vi "Fundamental Power Values (1 Cycle).vi"(0 "one-cycle fundamental phase voltage vectors":T3(array[cluster]), 5 "one-cycle fundamental current vectors":T3(array[cluster]), 9 "system info in":refnum<class "EP System Info.lvclass">, 11 "error in (no error)":errorcluster) -> (4 "one-cycle fundamental power values":T1(array[cluster]), 10 "system info out":refnum<class "EP System Info.lvclass">, 15 "error out":errorcluster)   [LabVIEW 2014, in "NI_EP_Power Quality.lvlib"]
doc: "Calculates the fundamental power values from the voltage and current spectra for a single-cycle block.\n\nThis VI supports measuring single-line and multiple-line systems."
uses:
  <vilib>/addons/Electrical Power/PQ/NI_EP_Power Quality.lvlib
  <vilib>/addons/Electrical Power/PQ/Common/Controls/ep_AI Data Channel.ctl
  <vilib>/addons/Electrical Power/PQ/Common/Classes/System Info/EP System Info.lvclass
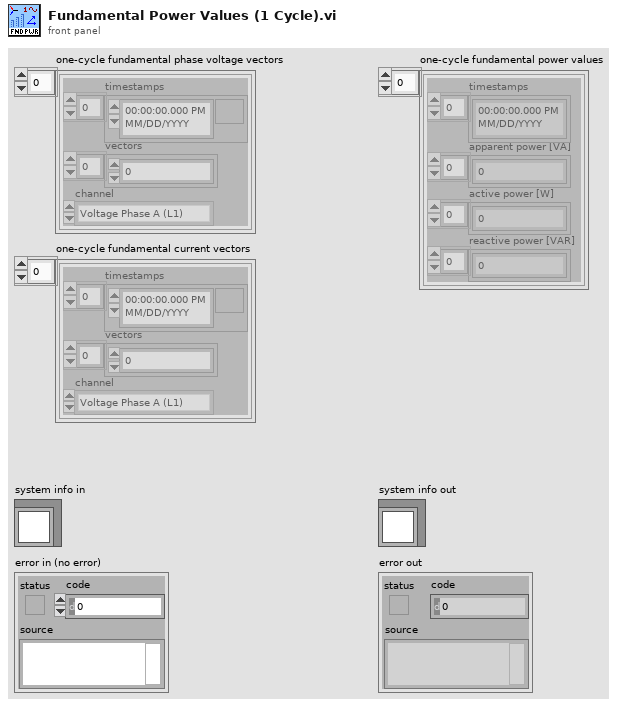
[diagram p1: front panel]
types:
  T1 = cluster{"timestamps":timestamp[], "apparent power [VA]":dbl[], "active power [W]":dbl[], "reactive power [VAR]":dbl[]}[]
  T2 = typedef "NI_EP_Power Quality.lvlib/ep_AI Data Channel.ctl" = enum16{"Voltage Phase A (L1)", "Voltage Phase B (L2)", "Voltage Phase C (L3)", "Voltage Phase N (Neutral)", "Current Phase A (L1)", "Current Phase B (L2)", "Current Phase C (L3)", "Current Phase N (Neutral)"}
  T3 = cluster{"timestamps":timestamp[], "vectors":cdb[], "channel":T2}[]
  T4 = cluster{"timestamps":timestamp[], dbl[], dbl[], dbl[]}
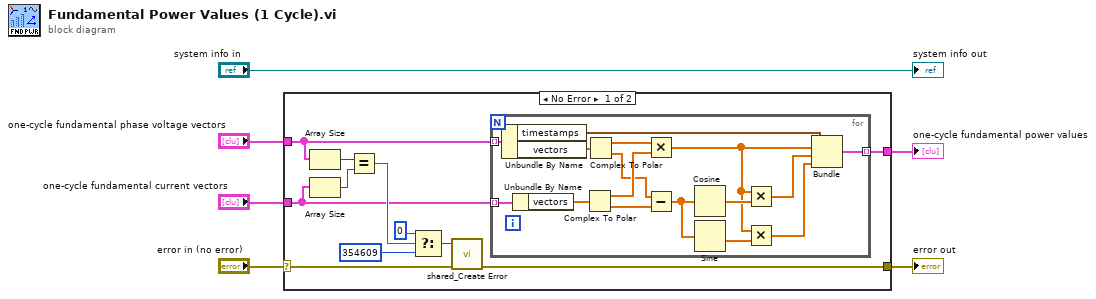
[diagram p0: block diagram]
diagram:
  n1 = case shown="No Error" "error in (no error)" {
    selector: "error in (no error)" -> [w8 w34]
    tunnel: "one-cycle fundamental phase voltage vectors" -> [w12 _]
    tunnel: "one-cycle fundamental current vectors" -> [w11 _]
    tunnel: [w17 _] -> w5
    tunnel: [w7 w34] -> w1
    frame No Error {
      n2 = Array Size(array=w12) -> (size(s)=w10:i32)
      n3 = Array Size(array=w11) -> (size(s)=w9:i32)
      n4 = Equal?(x=w10, y=w9) -> (x = y?=w13:bool)
      n5 = Select(t=0 ("error code (0)"), s=w13, f=354609 ("error code (0)")) -> (s? t:f=w14:i32)
      n6 = call <vilib>:"shared_Create Error.vi"("error in (no error)"=w8, "error code (0)"=w14) -> ("error out"=w7:errorcluster)  [unwired: 9 in]
      n7 = for {
        tunnel: w12 -> [w33] mode=indexing
        tunnel: w11 -> [w18] mode=indexing
        tunnel: [w19] -> w17 mode=indexing
        n8 = Unbundle By Name(w33) -> ("timestamps"=w23:timestamp[], "vectors"=w32:cdb[])
        n9 = Unbundle By Name(w18) -> ("vectors"=w31:cdb[])
        n10 = Complex To Polar(r * e^(i*theta)=w31) -> (r=w26:dbl[], theta=w25:dbl[])
        n11 = Complex To Polar(r * e^(i*theta)=w32) -> (r=w27:dbl[], theta=w24:dbl[])
        n12 = Multiply(x=w27, y=w26) -> (x*y=w22:dbl[])
        n13 = Subtract(x=w24, y=w25) -> (x-y=w29:dbl[])
        n14 = Cosine(x=w29) -> (cos(x)=w28:dbl[])
        n15 = Sine(x=w29) -> (sin(x)=w30:dbl[])
        n16 = Multiply(x=w22, y=w28) -> (x*y=w21:dbl[])
        n17 = Multiply(x=w22, y=w30) -> (x*y=w20:dbl[])
        n18 = Bundle("timestamps"=w23, w22, w21, w20) -> (w19:T4)  [unwired: 1 in]
      }
    }
    frame Error {
    }
  }
  "error out" <- w1
  "one-cycle fundamental power values" <- w5
  "system info out" <- "system info in"
